vi "add_compression_policy.vi"(7 "connection_reference":T1, 8 "error in (no error)":errorcluster, 9 "if_not_exists":bool, 10 "compression_interval":dbl=86400.0 format="%<%H:%M:%S%4u>t", 11 "hyper_table_name":string) -> (0 "error out":errorcluster)   [LabVIEW 2015, in "lv-timescaledb.lvlib"]
uses:
  lv-timescaledb.lvlib
  <vilib>/addons/database/Connection.llb/Conn ObjectReference.ctl
  <vilib>/addons/database/Command.llb/Cmd Execute.vi
  <vilib>/addons/database/Recordset.llb/Rec Destroy - Command.vi
  <vilib>/addons/database/Command.llb/Cmd Delete.vi
  <vilib>/addons/database/NI_Database_API.lvlib
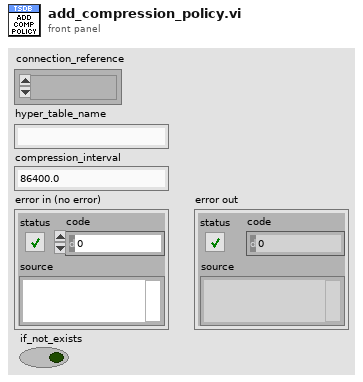
[diagram p1: front panel]
types:
  T1 = typedef "NI_Database_API.lvlib/Conn ObjectReference.ctl" = refnum<k1>
  T2 = cluster{"hyper_table_name":string, "if_not_exists":bool, "interval":string}
  T3 = typedef "NI_Database_API.lvlib/DB Tools Parameter Info.ctl" = cluster{"parameter name":string, "type":T4, "direction":T5, "value":variant}
  T4 = typedef "NI_Database_API.lvlib/DB Tools DataTypes.ctl" = enum16{"String", "Long (I32)", "Single (SGL)", "Double (DBL)", "Date/Time", "Binary"}
  T5 = typedef "NI_Database_API.lvlib/DB Tools Parameter Dir.ctl" = enum32{"Input", "Output", "Input/Output", "Return Value"}
  T6 = typedef "NI_Database_API.lvlib/Cmd ObjectReference.ctl" = refnum<k1>
  T7 = typedef "NI_Database_API.lvlib/Cmd-Rec Object Reference.ctl" = refnum<k1>
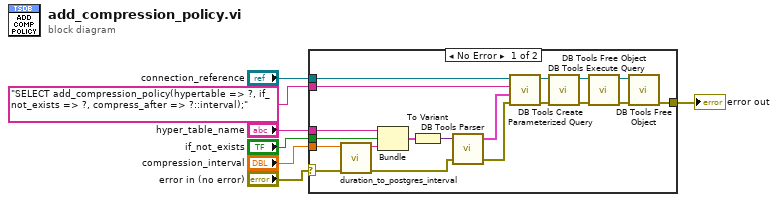
[diagram p0: block diagram]
diagram:
  n1 = case shown="No Error" "error in (no error)" {
    selector: "error in (no error)" -> [w8 w27]
    tunnel: "hyper_table_name" -> [w26 _]
    tunnel: "connection_reference" -> [w25 _]
    tunnel: [w24 w27] -> w5
    tunnel: "SELECT add_compression_policy(hypertable => ?, if_not_exists => ?, compress_after => ?::interval);" -> [w23 _]
    tunnel: "compression_interval" -> [w22 _]
    tunnel: "if_not_exists" -> [w21 _]
    frame No Error {
      n2 = call "duration_to_postgres_interval.vi"("error in (no error)"=w8, "relative_time"=w22) -> ("error out"=w10:errorcluster, "interval"=w9:string)  [unwired: 8 in]
      n3 = Bundle("hyper_table_name"=w26, "if_not_exists"=w21, "interval"=w9) -> (w14:T2)  [unwired: 1 in]
      n4 = To Variant(anything=w14) -> (Variant=w11:variant)
      n5 = call <vilib>:"DB Tools Parser.vi"("error in (no error)"=w10, "variant"=w11) -> ("error out"=w12:errorcluster, "parameters"=w13:T3[])  [unwired: 2 in]
      n6 = call <vilib>:"DB Tools Create Parameterized Query.vi"("error in (no error)"=w12, "parameters"=w13, "SQL query"=w23, "connection reference"=w25) -> ("error out"=w19:errorcluster, "command reference"=w17:T6)  [unwired: 3 in, 1 out]
      n7 = call-poly <vilib>:"DB Tools Execute Query.vi"("error in (no error)"=w19, "command reference"=w17) -> ("error out"=w20:errorcluster, "command-recordset reference"=w16:T7)  [unwired: 6 in]
      n8 = call-poly <vilib>:"DB Tools Free Object.vi"("error in (no error)"=w20, "command-recordset reference"=w16) -> ("error out"=w18:errorcluster, "command reference"=w15:T6)  [unwired: 8 in]
      n9 = call-poly <vilib>:"DB Tools Free Object.vi"("error in (no error)"=w18, "command reference"=w15) -> ("error out"=w24:errorcluster)  [unwired: 8 in, 1 out]
    }
    frame Error {
    }
  }
  "error out" <- w5
